vi "open camera settings.vi"(8 "error in (no error)":errorcluster, 11 "IMAQdx Actor in":refnum<class "IMAQdx Actor.lvclass">) -> (0 "error out":errorcluster, 3 "IMAQdx Actor out":refnum<class "IMAQdx Actor.lvclass">)   [LabVIEW 2014, in "IMAQdx Actor.lvlib" / "IMAQdx Actor.lvclass"]
uses:
  IMAQdx Actor.lvclass
  Camera Settings Dialog/Camera Settings Dialog/Camera Settings Dialog.lvclass
  IMAQdx Actor.lvclass/IMAQdx Actor.ctl
  Camera Settings Dialog/Camera Settings Dialog/Camera Settings Dialog.lvclass/Camera Settings Dialog.ctl
  <vilib>/ActorFramework/Message Enqueuer/Message Enqueuer.lvclass/Message Enqueuer.ctl
  Camera Settings Dialog/Camera Settings Dialog/Write IMAQdx Session.vi
  <vilib>/ActorFramework/Message Enqueuer/Enqueue.vi
  <vilib>/ActorFramework/Message Priority Queue/Priority Enqueue.vi
  Viewable Actor/ViewableActor Messages/Open Front Panel Msg/Open Front Panel Msg.lvclass
  <vilib>/ActorFramework/Actor/Actor.lvclass
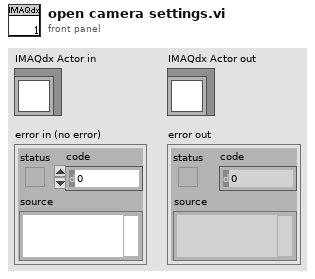
[diagram p1: front panel]
types:
  T1 = typedef "IMAQdx.ctl" = refnum<k21>
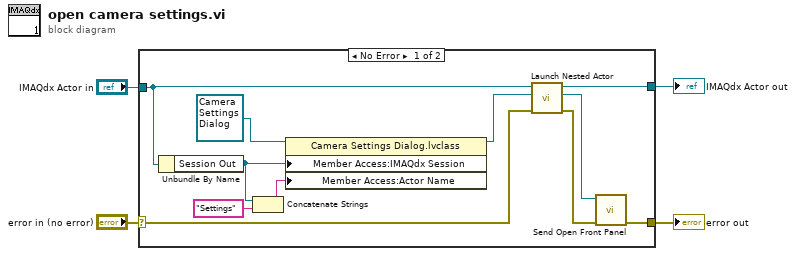
[diagram p0: block diagram]
diagram:
  n1 = case shown="No Error" "error in (no error)" {
    selector: "error in (no error)" -> [w11 w17]
    tunnel: [w8 w17] -> w3
    tunnel: [w15 w16] -> w1
    tunnel: "IMAQdx Actor in" -> [w12 w16]
    frame No Error {
      n2 = Unbundle By Name(w12) -> ("Session Out"=w6:T1)
      n3 = Concatenate Strings(w6, "Settings" ("string")) -> (w7:string)
      n4 = property class="Camera Settings Dialog.lvclass"(reference=refnum<class "Camera Settings Dialog.lvclass"> refnum ("Camera Settings Dialog.lvlib:Camera Settings Dialog.lvclass"), "Member Access:IMAQdx Session"=w6, "Member Access:Actor Name"=w7) -> (reference out=w13:refnum<class "Camera Settings Dialog.lvclass">)  [unwired: 1 in, 1 out]
      n5 = call <vilib>:"Launch Nested Actor.vi"("error in (no error)"=w11, "Nested Actor"=w13, "Caller Actor in"=w12) -> ("error out"=w9:errorcluster, "Nested Actor's Enqueuer"=w10:refnum<class "Message Enqueuer.lvclass">, "Caller Actor out"=w15:refnum<class "IMAQdx Actor.lvclass">)  [unwired: 6 in]
      n6 = call "Send Open Front Panel.vi"("error in (no error)"=w9, "Message Enqueuer"=w10) -> ("error out"=w8:errorcluster)  [unwired: 8 in, 1 out]
    }
    frame Error {
    }
  }
  "error out" <- w3
  "IMAQdx Actor out" <- w1
